vi "send relative move to stage.vi"(8 "error in (no error)":errorcluster, 10 "relative move to send":dbl, 11 "Thorcam in":refnum<class "Thorcam.lvclass">) -> (0 "error out":errorcluster, 3 "Thorcam out":refnum<class "Thorcam.lvclass">)   [LabVIEW 2012, in "Thorcam.lvclass"]
uses:
  Thorcam.lvclass
  <vilib>/Distrio/Murmex/GenericMessage/GenericMessage.lvclass
  Thorcam.lvclass/Thorcam.ctl
  <vilib>/Distrio/Murmex/Message/Message.lvclass
  <vilib>/Distrio/Murmex/Murmex/Murmex.lvclass
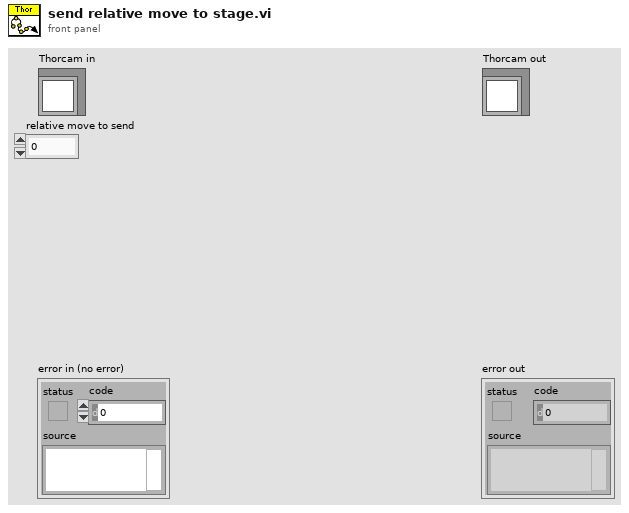
[diagram p1: front panel]
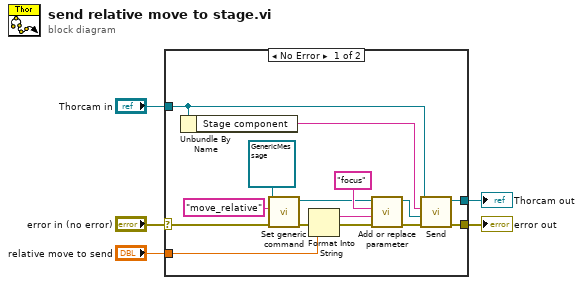
[diagram p0: block diagram]
diagram:
  n1 = case shown="No Error" "error in (no error)" {
    selector: "error in (no error)" -> [w18 w22]
    tunnel: [w12 w22] -> w4
    tunnel: [w10 w21] -> w2
    tunnel: "Thorcam in" -> [w7 w21]
    tunnel: "relative move to send" -> [w9 _]
    frame No Error {
      n2 = Unbundle By Name(w7) -> ("Stage component"=w6:string)
      n3 = call <vilib>:"Set generic command.vi"("error in (no error)"=w18, "generic command"="move_relative" ("command string"), "GenericMessage in"=refnum<class "GenericMessage.lvclass"> refnum ("Murmex.lvlib:GenericMessage")) -> ("error out"=w14:errorcluster, "GenericMessage out"=w8:refnum<class "GenericMessage.lvclass">)  [unwired: 7 in]
      n4 = Format Into String(error in=w14, w9) -> (resulting string=w16:string, error out=w15:errorcluster)  [unwired: 2 in]
      n5 = call <vilib>:"Add or replace parameter.vi"("error in (no error)"=w15, "value"=w16, "name"="focus", "Message in"=w8) -> ("error out"=w13:errorcluster, "Message out"=w11:refnum<class "GenericMessage.lvclass">)  [unwired: 6 in]
      n6 = call <vilib>:"Send.vi"("error in (no error)"=w13, "Message"=w11, "recipient"=w6, "Murmex in"=w7) -> ("error out"=w12:errorcluster, "Murmex out"=w10:refnum<class "Thorcam.lvclass">)  [unwired: 6 in]
    }
    frame Error {
    }
  }
  "error out" <- w4
  "Thorcam out" <- w2
